vi "Shutdown.vi"(8 "error in (no error)":errorcluster, 11 "DAQ_Engine in":refnum<class "DAQ_Engine.lvclass">) -> (0 "error out":errorcluster, 3 "DAQ_Engine out":refnum<class "DAQ_Engine.lvclass">)   [LabVIEW 2019, in "DAQ_Engine.lvclass"]
doc: "Developed by Kevin Thompson\nkevin@thompsonengineering.net\n\nCopyright 2018\nThompson Engineering, LLC"
uses:
  DAQ_Engine.lvclass
  DAQ_Engine.lvclass/DAQ_Engine.ctl
  Accessors/Get Settings.vi
  Config/Accessors/Set DAQ Settings.vi
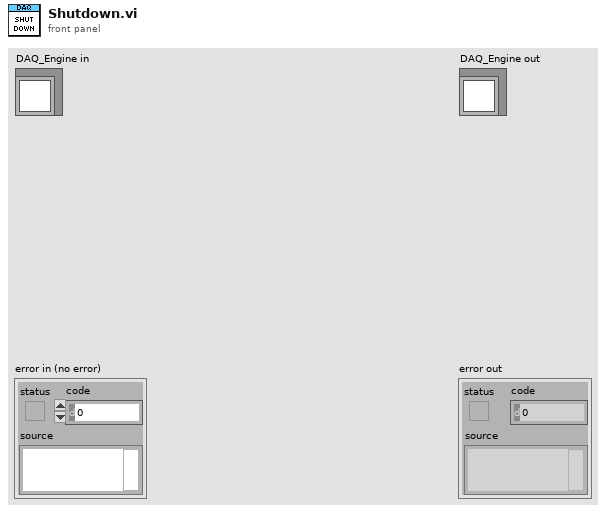
[diagram p1: front panel]
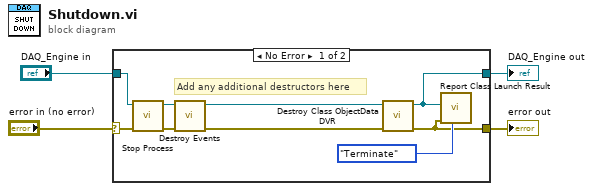
[diagram p0: block diagram]
diagram:
  n1 = case shown="No Error" "error in (no error)" {
    selector: "error in (no error)" -> [w5 w15]
    tunnel: [w7 w15] -> w3
    tunnel: [w8 w14] -> w1
    tunnel: "DAQ_Engine in" -> [w6 w14]
    frame No Error {
      # "Add any additional destructors here"
      n2 = call "Stop Process.vi"("error in (no error)"=w5, "DAQ_Engine in"=w6) -> ("error out"=w13:errorcluster, "DAQ_Engine out"=w12:refnum<class "DAQ_Engine.lvclass">)  [unwired: 8 in]
      n3 = call "Destroy Events.vi"("error in (no error)"=w13, "DAQ_Engine in"=w12) -> ("error out"=w11:errorcluster, "DAQ_Engine out"=w10:refnum<class "DAQ_Engine.lvclass">)  [unwired: 8 in]
      n4 = call "Destroy Class ObjectData DVR.vi"("error in (no error)"=w11, "DAQ_Engine in"=w10) -> ("error out"=w7:errorcluster, "DAQ_Engine out"=w8:refnum<class "DAQ_Engine.lvclass">)  [unwired: 8 in]
      n5 = call "Report Class Launch Result.vi"("Object"=w8, "error in (no error)"=w7, "Mode (Launch)"=enum16{"Launch", "Terminate"}."Terminate") -> ()  [unwired: 7 in, 1 out]
    }
    frame Error {
    }
  }
  "error out" <- w3
  "DAQ_Engine out" <- w1
